vi "FalloutControlArmInterfaceUSB.vi"() -> ()   [LabVIEW 2024]
uses:
  <vilib>/Instr/_visa.llb/VISA Configure Serial Port (Instr).vi
panel:
  out "concatenated string 2":string
  out "concatenated string":string
  in  "Power Button":bool
  in  "Position Maximum":bool
  in  "Position Minimum":bool
  in  "BackwardButton":bool
  in  "ForwardButton":bool
  in  "ScramButton":bool
  in  "SpeedSelectButton":bool
  in  "ElectormagnetButton":bool
  out "Analog In 4":u16(slide)=187 scale=0.0..1023.0
  out "Analog In 3":u16(slide)=187 scale=0.0..1023.0
  out "Analog In 2":u16(slide)=187 scale=0.0..1023.0
  out "Analog In 1":u16(slide)=187 scale=0.0..1023.0
  out "Digital Inputs 2":bool[](array[boolean])=[TRUE, TRUE, TRUE, TRUE, TRUE, TRUE, TRUE, TRUE]
  out "Digital Inputs":bool[](array[boolean])=[TRUE, TRUE, TRUE, TRUE, TRUE, TRUE, TRUE, TRUE]
  out "Hex data received":string
  in  "stop":bool
  in  "VISA resource name":refnum<visa-resource-name>
  # "Analog Inputs"
  # "Digital Indicators"
  # "Debug Section"
  # "Motor Active"
  # "Scram Bit\nPower Bit\nMagnet Bit\nForward Bit\nBackward Bit\nMinimum Position \nMaximum Position\nSpeed Select Bit"
  # "Digital Buttons"
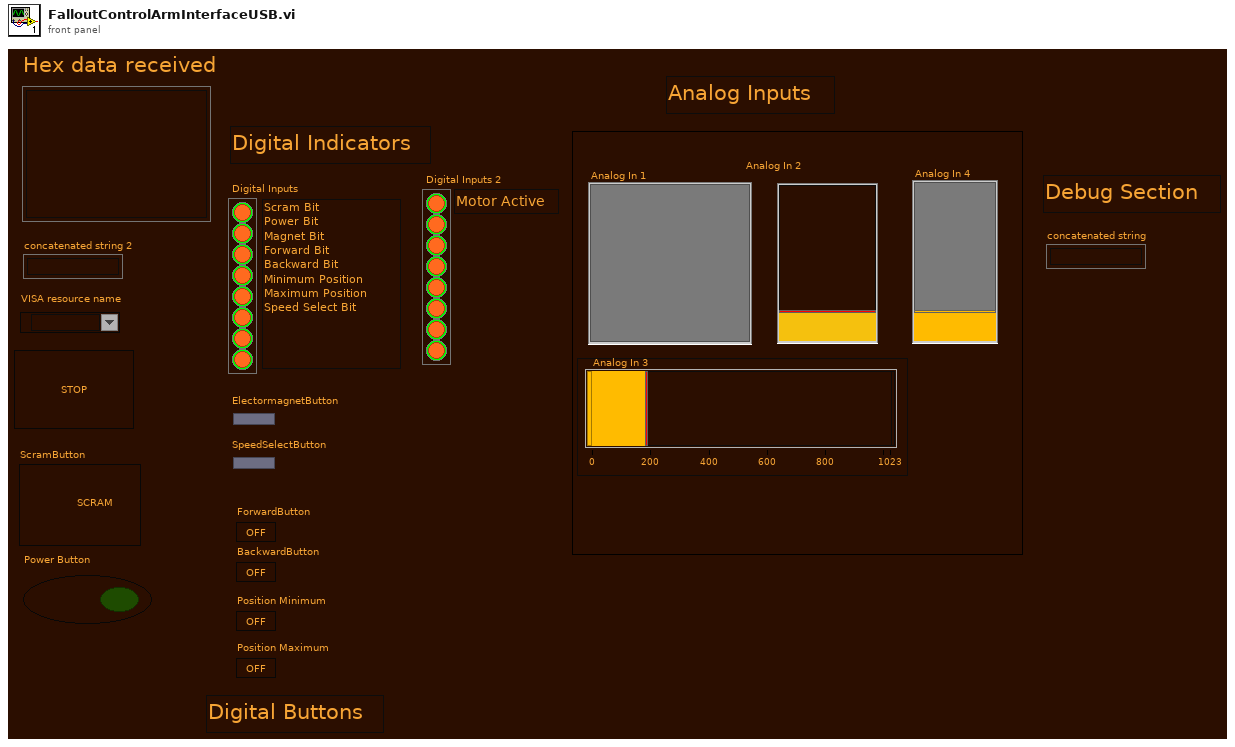
[diagram p1: front panel]
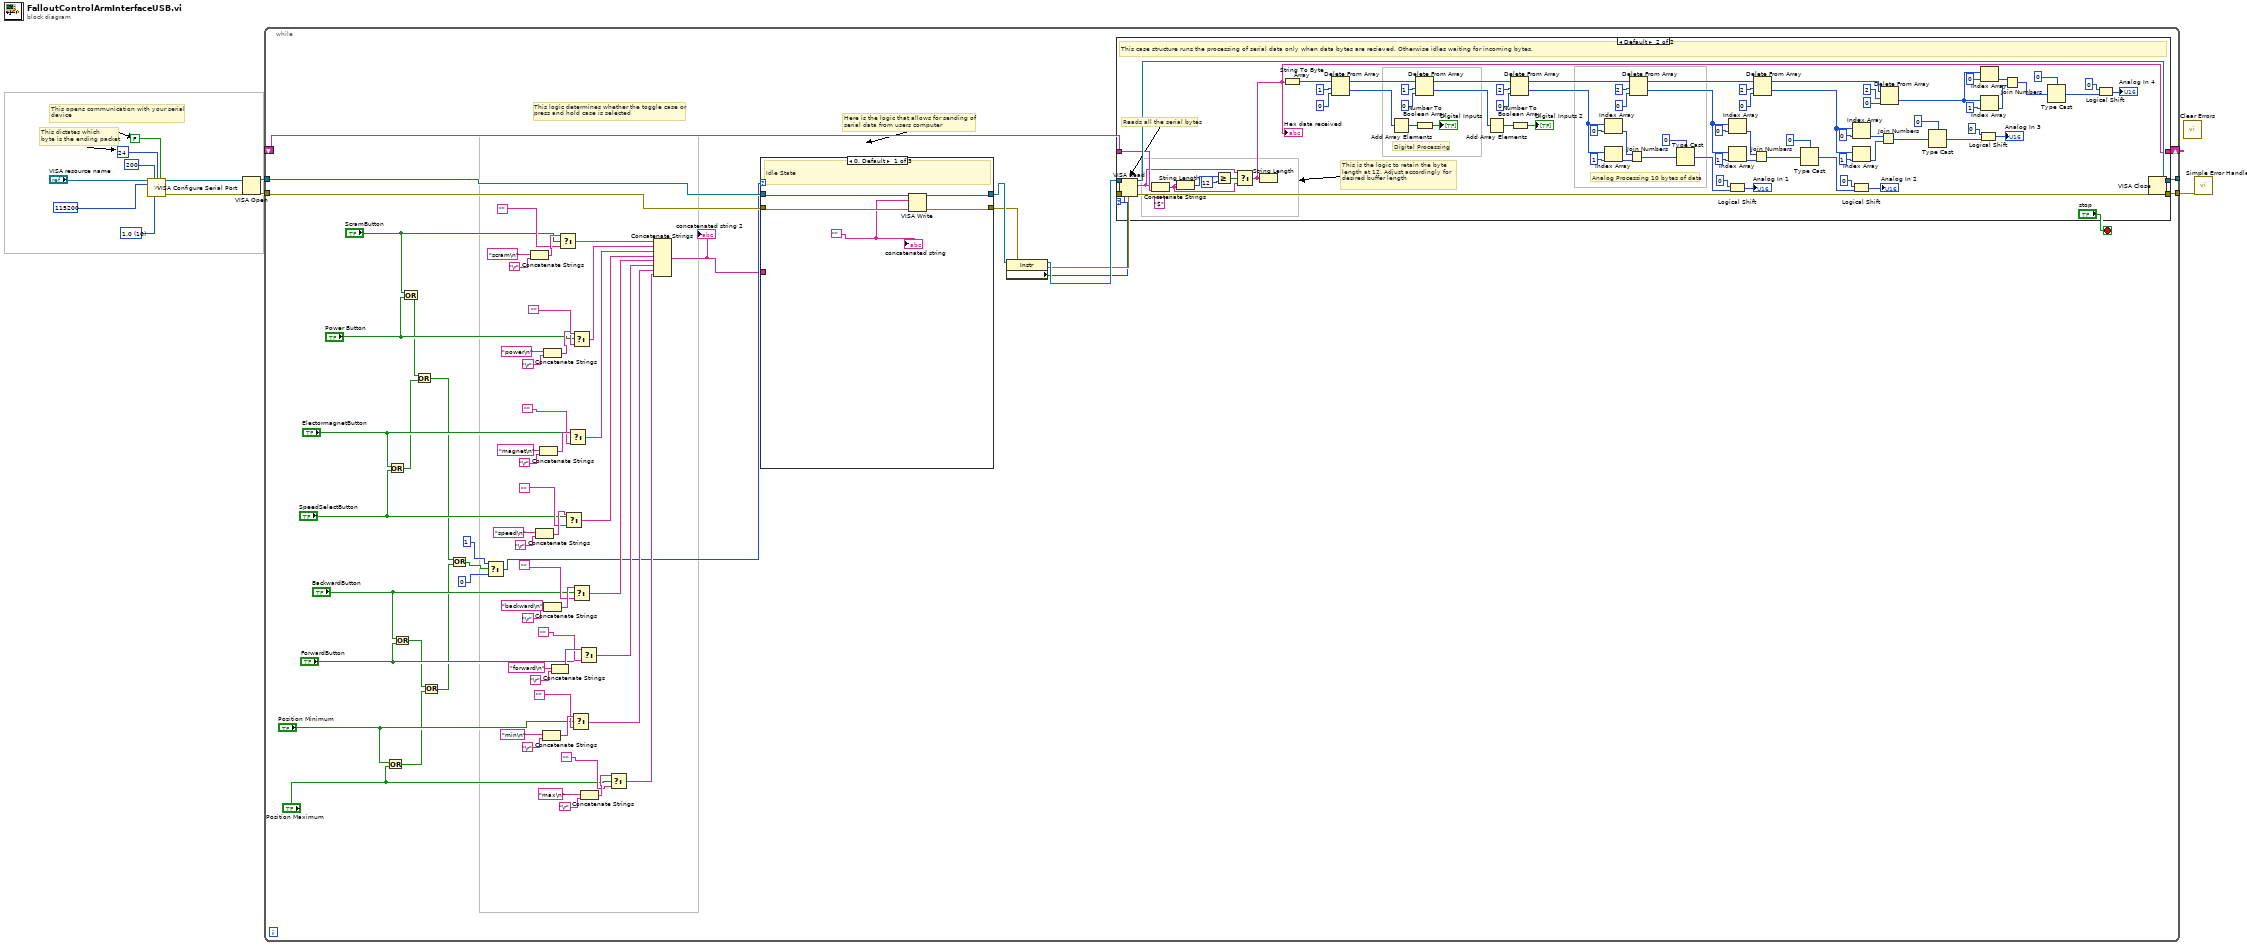
[diagram p0: block diagram]
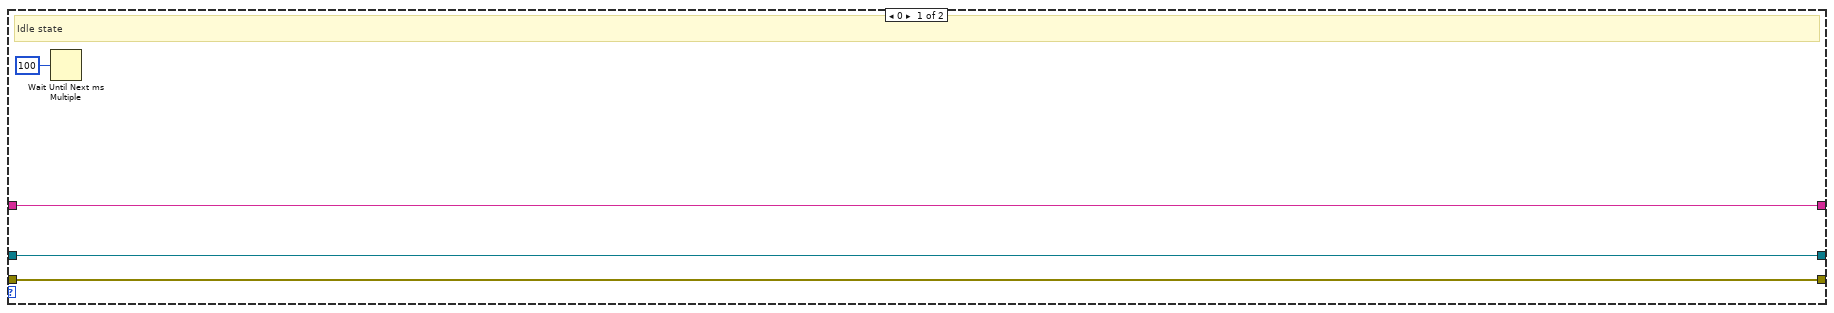
[diagram p2: hidden frame]
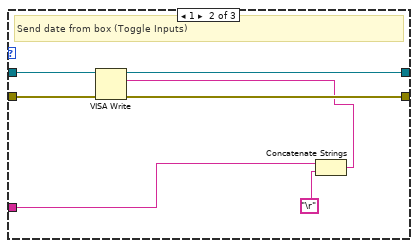
[diagram p3: hidden frame]
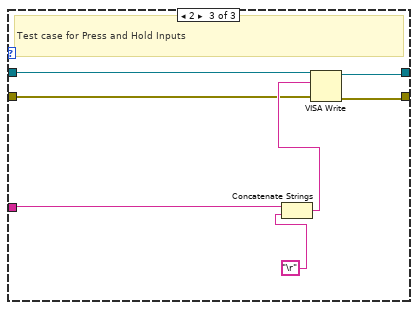
[diagram p4: hidden frame]
diagram:
  w6 = u16 10 items=["1.0"=10, "1.5"=15, "2.0"=20] ("stop bits (10: 1 bit)")
  # "This dictates which\nbyte is the ending packet"
  # "This opens communication with your serial\ndevice"
  n1 = call-poly "VISA Configure Serial Port"("VISA resource name"="VISA resource name", "timeout (10sec)"=u32 200, "termination char\n(0xA = '\\n' = LF)"=u8 24 ("termination char\n(0xA = '\\n' = LF)"), "Enable Termination\nChar (T)"=FALSE ("Enable Termination\nChar (T)"), "baud rate (9600)"=u32 115200, "stop bits (10: 1 bit)"=w6) -> ("VISA resource name out"=w2:refnum<visa-resource-name>, "error out"=w1:errorcluster)  [unwired: 8 in]
  n2 = VISA Open(error in (no error)=w1, VISA resource name=w2) -> (VISA resource name=w9:refnum<visa-resource-name>, error out=w8:errorcluster)  [unwired: 3 in]
  n3 = while {
    shift-right: [w78] -> _
    shift-left: _ -> [w77]
    tunnel: w9 -> [w76]
    tunnel: w8 -> [w75]
    tunnel: [w74] -> w4
    tunnel: [w73] -> w3
    stop <- "stop" stop-if-true
    # "This logic determines whether the toggle case or \npress and hold case is selected"
    # "Here is the logic that allows for sending of \nserial data from users computer"
    n4 = Or(x="Position Minimum", y="Position Maximum") -> (x .or. y?=w24:bool)
    n5 = Or(x="ElectormagnetButton", y="SpeedSelectButton") -> (x .or. y?=w22:bool)
    n6 = Or(x="BackwardButton", y="ForwardButton") -> (x .or. y?=w23:bool)
    n7 = Or(x="ScramButton", y="Power Button") -> (x .or. y?=w21:bool)
    n8 = Or(x=w21, y=w22) -> (x .or. y?=w20:bool)
    n9 = Or(x=w23, y=w24) -> (x .or. y?=w19:bool)
    n10 = Or(x=w20, y=w19) -> (x .or. y?=w18:bool)
    n11 = Select(t=1, s=w18, f=0) -> (s? t:f=w15:i32)
    n12 = Concatenate Strings("scram\n", "\r") -> (w48:string)
    n13 = Concatenate Strings("speed\n", "\r") -> (w45:string)
    n14 = Concatenate Strings("magnet\n", "\r") -> (w46:string)
    n15 = Concatenate Strings("min\n", "\r") -> (w42:string)
    n16 = Concatenate Strings("power\n", "\r") -> (w47:string)
    n17 = Concatenate Strings("backward\n", "\r") -> (w44:string)
    n18 = Concatenate Strings("forward\n", "\r") -> (w43:string)
    n19 = Select(t=w48, s="ScramButton", f="") -> (s? t:f=w56:string)
    n20 = Select(t=w45, s="SpeedSelectButton", f="") -> (s? t:f=w53:string)
    n21 = Select(t=w46, s="ElectormagnetButton", f="") -> (s? t:f=w54:string)
    n22 = Select(t=w42, s="Position Minimum", f="") -> (s? t:f=w50:string)
    n23 = Select(t=w47, s="Power Button", f="") -> (s? t:f=w55:string)
    n24 = Select(t=w44, s="BackwardButton", f="") -> (s? t:f=w52:string)
    n25 = Select(t=w43, s="ForwardButton", f="") -> (s? t:f=w51:string)
    n26 = Concatenate Strings("max\n", "\r") -> (w41:string)
    n27 = Select(t=w41, s="Position Maximum", f="") -> (s? t:f=w49:string)
    n28 = Concatenate Strings(w56, w55, w54, w53, w52, w51, w50, w49) -> (w14:string)
    "concatenated string 2" <- w14
    n29 = case shown="0, Default" w15 {
      tunnel: [w168 w176 w181] -> w82
      tunnel: w76 -> [w167 w175 w180]
      tunnel: w75 -> [w166 w174 w179]
      tunnel: [w169 w173 w182] -> w83
      tunnel: w14 -> [_ w170 w177]
      frame 0, Default {
        w165 = ""
        # "Idle State"
        n30 = VISA Write(VISA resource name=w167, write buffer=w165, error in (no error)=w166) -> (VISA resource name out=w169:refnum<visa-resource-name>, error out=w168:errorcluster)  [unwired: 1 out]
        "concatenated string" <- w165
      }
      frame 1 {
        # "Send date from box (Toggle Inputs)"
        n31 = Concatenate Strings "Concatenate Strings"(w170, "\r") -> (w172:string)
        n32 = VISA Write(VISA resource name=w175, write buffer=w172, error in (no error)=w174) -> (VISA resource name out=w173:refnum<visa-resource-name>, error out=w176:errorcluster)  [unwired: 1 out]
      }
      frame 2 {
        # "Test case for Press and Hold Inputs"
        n33 = Concatenate Strings "Concatenate Strings"(w177, "\r") -> (w183:string)
        n34 = VISA Write(VISA resource name=w180, write buffer=w183, error in (no error)=w179) -> (VISA resource name out=w182:refnum<visa-resource-name>, error out=w181:errorcluster)  [unwired: 1 out]
      }
    }
    n35 = property class="Instr"(reference=w83, error in=w82) -> (reference out=w81:refnum<visa-resource-name>, error out=w80:errorcluster, "Serial Settings:Number of Bytes at Serial Port"=w79:u32)
    n36 = case shown="Default" w79 {
      selector: w79 -> [_ w160]
      tunnel: [w88 w164] -> w73
      tunnel: [w87 w163] -> w74
      tunnel: w81 -> [w88 w162]
      tunnel: w80 -> [w87 w161]
      tunnel: w77 -> [w85 w159]
      tunnel: [w85 w147] -> w78
      frame 0 {
        # "Idle state"
        n37 = Wait Until Next ms Multiple(millisecond multiple=u32 100 ("millisecond timer value")) -> ()  [unwired: 1 out]
      }
      frame Default {
        (unwired) "$"
        # "Analog Processing 10 bytes of data"
        # "Digital Processing"
        # "This is the logic to retain the byte length at 12. Adjust accordingly for \ndesired buffer length"
        # "Reads all the serial bytes"
        # "This case structure runs the processing of serial data only when data bytes are recieved. Otherwise idles waiting for incoming bytes."
        n38 = VISA Read(VISA resource name=w162, byte count=w160, error in (no error)=w161) -> (VISA resource name out=w164:refnum<visa-resource-name>, read buffer=w155:string, error out=w163:errorcluster)  [unwired: 1 out]
        n39 = Concatenate Strings(w155, w159) -> (w154:string)
        n40 = String Length(string=w154) -> (length=w158:i32)
        n41 = Greater Or Equal?(x=w158, y=12) -> (x >= y?=w156:bool)
        n42 = Select(t=w155, s=w156, f=w154) -> (s? t:f=w147:string)
        "Hex data received" <- w147
        n43 = String Length(string=w147) -> ()  [unwired: 1 out]
        n44 = String To Byte Array(string=w147) -> (unsigned byte array=w152:u8[])
        n45 = Delete From Array "Delete From Array"(array=w152, length=1, index=0) -> (deleted portion=w153:u8[], array with subset deleted=w143:u8[])
        n46 = Add Array Elements(numeric array=w153) -> (sum=w151:u8)
        n47 = Delete From Array "Delete From Array"(array=w143, length=1, index=0) -> (deleted portion=w144:u8[], array with subset deleted=w93:u8[])
        n48 = Number To Boolean Array(number=w151) -> (Boolean array=→"Digital Inputs":bool[])
        n49 = Add Array Elements(numeric array=w144) -> (sum=w141:u8)
        n50 = Delete From Array "Delete From Array"(array=w93, length=2, index=0) -> (deleted portion=w134:u8[], array with subset deleted=w92:u8[])
        n51 = Number To Boolean Array(number=w141) -> (Boolean array=→"Digital Inputs 2":bool[])
        n52 = Index Array(array=w134, index=0) -> (element=w131:u8)
        n53 = Index Array(array=w134, index=1) -> (element=w130:u8)
        n54 = Join Numbers(hi=w131, lo=w130) -> ((hi.lo)=w129:u16)
        n55 = Delete From Array "Delete From Array"(array=w92, length=2, index=0) -> (deleted portion=w123:u8[], array with subset deleted=w91:u8[])
        n56 = Type Cast(type=u16 0 ("y"), x=w129) -> (*(type *) &x=w138:u16)
        n57 = Logical Shift(y=i16 0, x=w138) -> (x << y=→"Analog In 1":u16)
        n58 = Index Array(array=w123, index=0) -> (element=w126:u8)
        n59 = Index Array(array=w123, index=1) -> (element=w127:u8)
        n60 = Join Numbers(hi=w126, lo=w127) -> ((hi.lo)=w128:u16)
        n61 = Delete From Array "Delete From Array"(array=w91, length=2, index=0) -> (deleted portion=w110:u8[], array with subset deleted=w90:u8[])
        n62 = Type Cast(type=u16 0 ("y"), x=w128) -> (*(type *) &x=w119:u16)
        n63 = Logical Shift(y=i16 0, x=w119) -> (x << y=→"Analog In 2":u16)
        n64 = Index Array(array=w110, index=0) -> (element=w107:u8)
        n65 = Index Array(array=w110, index=1) -> (element=w106:u8)
        n66 = Join Numbers(hi=w107, lo=w106) -> ((hi.lo)=w105:u16)
        n67 = Delete From Array "Delete From Array"(array=w90, length=2, index=0) -> (deleted portion=w100:u8[])  [unwired: 1 out]
        n68 = Type Cast(type=u16 0 ("y"), x=w105) -> (*(type *) &x=w114:u16)
        n69 = Logical Shift(y=i16 0, x=w114) -> (x << y=→"Analog In 3":u16)
        n70 = Index Array(array=w100, index=0) -> (element=w102:u8)
        n71 = Index Array(array=w100, index=1) -> (element=w103:u8)
        n72 = Join Numbers(hi=w102, lo=w103) -> ((hi.lo)=w104:u16)
        n73 = Type Cast(type=u16 0 ("y"), x=w104) -> (*(type *) &x=w96:u16)
        n74 = Logical Shift(y=i16 0, x=w96) -> (x << y=→"Analog In 4":u16)
      }
    }
  }
  n75 = VISA Close(VISA resource name=w3, error in (no error)=w4) -> (error out=w5:errorcluster)
  n76 = call <vilib>:"Clear Errors.vi"() -> ()  [unwired: 6 in, 2 out]
  n77 = call <vilib>:"Simple Error Handler.vi"("error in (no error)"=w5) -> ()  [unwired: 4 in, 5 out]
